vi "Clear Specific Error.vi"(8 "error in":errorcluster, 10 "Code (-1:All)":i32=-1) -> (0 "error out":errorcluster, 2 "Error Cleared":bool)   [LabVIEW 2013, in "Mercury iXX.lvlib"]
uses:
  <instrlib>/Mercury iXX/Mercury iXX.lvlib
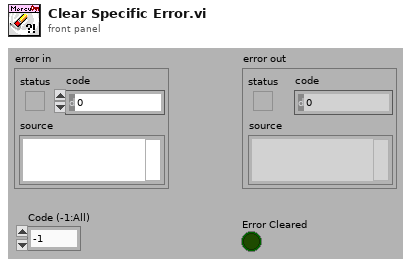
[diagram p1: front panel]
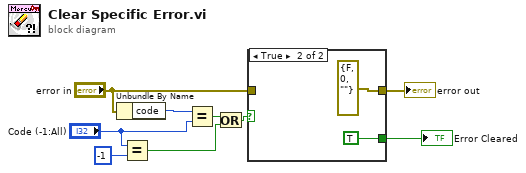
[diagram p0: block diagram]
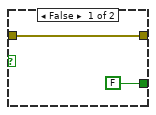
[diagram p2: hidden frame]
diagram:
  n1 = Unbundle By Name("error in") -> ("code"=w9:i32)
  n2 = Equal?(x="Code (-1:All)", y=-1 ("x")) -> (x = y?=w2:bool)
  n3 = Equal?(x=w9, y="Code (-1:All)") -> (x = y?=w8:bool)
  n4 = Or(x=w8, y=w2) -> (x .or. y?=w3:bool)
  n5 = case shown="True" w3 {
    tunnel: "error in" -> [w11 _]
    tunnel: [w11 errorcluster {"status"=FALSE, "code"=0, "source"=""} ("error in (no error)")] -> w6
    tunnel: [FALSE ("status") TRUE ("status")] -> w5
    frame False {
    }
    frame True {
    }
  }
  "error out" <- w6
  "Error Cleared" <- w5
